vi "scan_operation.vi"(4 "Iter Counter In":u16[](array[numeric]), 5 "Prev DIO State":bool[](array[boolean])=[FALSE, FALSE, FALSE, FALSE, FALSE, FALSE, FALSE, FALSE, FALSE, FALSE, FALSE, FALSE, FALSE, FALSE, FALSE, FALSE, FALSE, FALSE, FALSE, FALSE, FALSE, FALSE, FALSE, FALSE, FALSE, FALSE, FALSE, FALSE, FALSE, FALSE, FALSE, FALSE], 6 "Digital Input Value Array":bool[](array[boolean])=[FALSE, FALSE, FALSE, FALSE, FALSE, FALSE, FALSE, FALSE, FALSE, FALSE, FALSE, FALSE, FALSE, FALSE, FALSE, FALSE, FALSE, FALSE, FALSE, FALSE, FALSE, FALSE, FALSE, FALSE, FALSE, FALSE, FALSE, FALSE, FALSE, FALSE, FALSE, FALSE], 7 "Channel":T1={"Operation"=0, "Num. Steps"=0, "Begin"=0.0, "Step Size"=0.0, "Input - A"=0, "Input - B"=0, "Output - LO"=0.0, "Output - HI"=0.0, "Reset"=FALSE, "Analog Output"=0, "Trigger Input"=0, "Initialize To"=0, "Digital Inputs"=[0, 0, 0, 0, 0], "Output Values"=[0.0, 0.0, 0.0, 0.0, 0.0], "Num. Inputs"=4} {"Digital Inputs" items=["DIO0", "DIO1", "DIO2", "DIO3", "DIO4", "DIO5", "DIO6", "DIO7", "DIO8", "DIO9", "DIO10", "DIO11", "DIO12", "DIO13", "DIO14", "DIO15", "DIO16", "DIO17", "DIO18", "DIO19", "DIO20", "DIO21", "DIO22", "DIO23", "DIO24", "DIO25", "DIO26", "DIO27", "DIO28", "DIO29", "DIO30", "DIO31"]; "Initialize To" items=["Zero", "Begin Value"]; "Trigger Input" items=["DIO0", "DIO1", "DIO2", "DIO3", "DIO4", "DIO5", "DIO6", "DIO7", "DIO8", "DIO9", "DIO10", "DIO11", "DIO12", "DIO13", "DIO14", "DIO15", "DIO16", "DIO17", "DIO18", "DIO19", "DIO20", "DIO21", "DIO22", "DIO23", "DIO24", "DIO25", "DIO26", "DIO27", "DIO28", "DIO29", "DIO30", "DIO31"]; "Analog Output" items=["AO\\00", "AO\\01", "AO\\02", "AO\\03", "AO\\04", "AO\\05", "AO\\06", "AO\\07", "AO\\08", "AO\\09", "AO\\10", "AO\\11", "AO\\12", "AO\\13", "AO\\14", "AO\\15"]; "Input - B" items=["DIO0", "DIO1", "DIO2", "DIO3", "DIO4", "DIO5", "DIO6", "DIO7", "DIO8", "DIO9", "DIO10", "DIO11", "DIO12", "DIO13", "DIO14", "DIO15", "DIO16", "DIO17", "DIO18", "DIO19", "DIO20", "DIO21", "DIO22", "DIO23", "DIO24", "DIO25", "DIO26", "DIO27", "DIO28", "DIO29", "DIO30", "DIO31"]; "Input - A" items=["DIO0", "DIO1", "DIO2", "DIO3", "DIO4", "DIO5", "DIO6", "DIO7", "DIO8", "DIO9", "DIO10", "DIO11", "DIO12", "DIO13", "DIO14", "DIO15", "DIO16", "DIO17", "DIO18", "DIO19", "DIO20", "DIO21", "DIO22", "DIO23", "DIO24", "DIO25", "DIO26", "DIO27", "DIO28", "DIO29", "DIO30", "DIO31"]; "Operation" items=["OFF", "SWITCH", "AND GATE", "OR GATE", "ITERATION", "CUSTOM - 461nm Freq."]}) -> (0 "Iter Counter Out":u16[](array[numeric]), 1 "Current DIO State":bool[](array[boolean]), 3 "AO out":fxp<+/-,20,5>)   [LabVIEW 2016]
uses:
  fpga_array_element.ctl
panel:
  # "Boolean Operation Controls"
  # "Iteration Operation Controls"
  # "Custom Operation Controls"
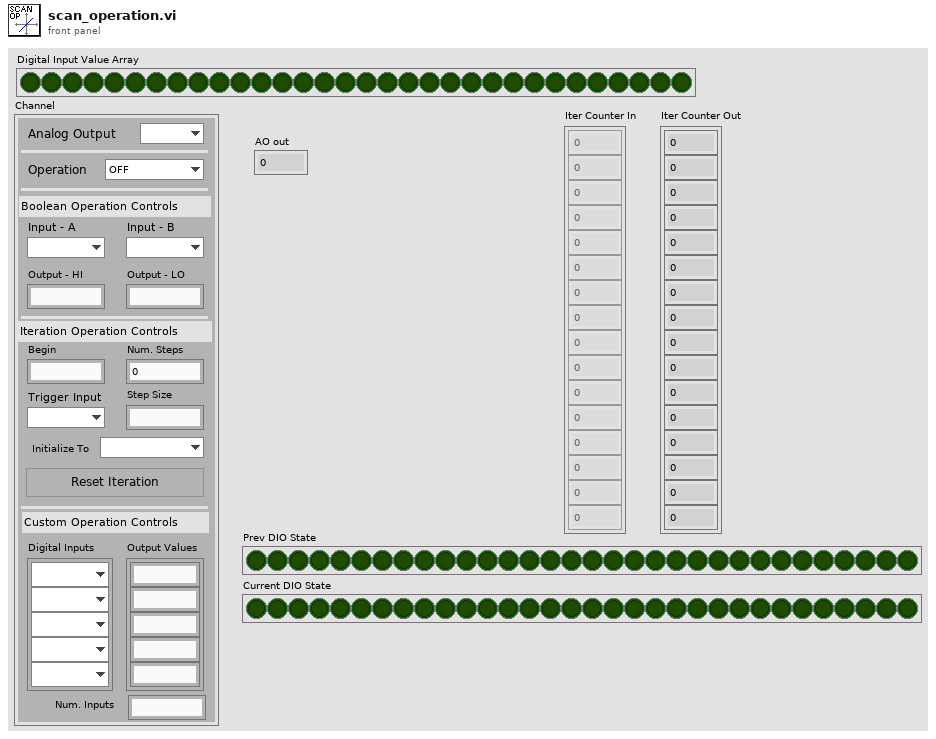
[diagram p1: front panel]
types:
  T1 = typedef "fpga_array_element.ctl" = cluster{"Operation":i16, "Num. Steps":u16, "Begin":fxp<+/-,20,5>, "Step Size":fxp<+/-,20,5>, "Input - A":i32, "Input - B":i32, "Output - LO":fxp<+/-,20,5>, "Output - HI":fxp<+/-,20,5>, "Reset":bool, "Analog Output":i32, "Trigger Input":i32, "Initialize To":i16, "Digital Inputs":i32[], "Output Values":fxp<+/-,20,5>[], "Num. Inputs":u16}
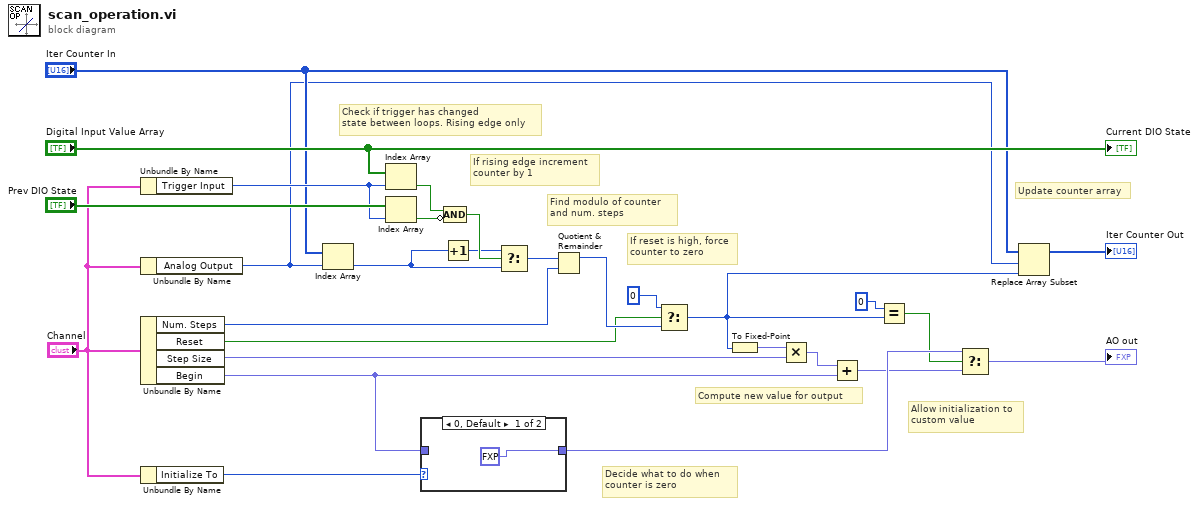
[diagram p0: block diagram]
diagram:
  # "Decide what to do when \ncounter is zero"
  # "Allow initialization to\ncustom value"
  # "Compute new value for output"
  # "Update counter array"
  # "If reset is high, force\ncounter to zero"
  # "Find modulo of counter\nand num. steps"
  # "If rising edge increment\ncounter by 1"
  # "Check if trigger has changed \nstate between loops. Rising edge only"
  n1 = Unbundle By Name("Channel") -> ("Trigger Input"=w24:i32)
  n2 = Unbundle By Name("Channel") -> ("Analog Output"=w1:i32)
  n3 = Unbundle By Name("Channel") -> ("Num. Steps"=w18:u16, "Reset"=w15:bool, "Step Size"=w14:fxp<+/-,20,5>, "Begin"=w10:fxp<+/-,20,5>)
  n4 = Unbundle By Name("Channel") -> ("Initialize To"=w11:i16)
  n5 = Index Array(array="Iter Counter In", index=w1) -> (element=w19:u16)
  n6 = Index Array(array="Digital Input Value Array", index=w24) -> (element=w26:bool)
  n7 = Index Array(array="Prev DIO State", index=w24) -> (element=w23:bool)
  n8 = case shown="0, Default" w11 {
    tunnel: w10 -> [_ w30]
    tunnel: [fxp<+/-,20,5> 0.0 w30] -> w7
    frame 0, Default {
    }
    frame 1 {
    }
  }
  n9 = Increment(x=w19) -> (x+1=w20:u16)
  n10 = Compound Arithmetic op=AND(w26, invert w23) -> (w28:bool)
  n11 = Select(t=w20, s=w28, f=w19) -> (s? t:f=w17:u16)
  n12 = Quotient & Remainder(x=w17, y=w18) -> (x-y*floor(x/y)=w16:u16)  [unwired: 1 out]
  n13 = Select(t=u16 0, s=w15, f=w16) -> (s? t:f=w9:u16)
  n14 = To Fixed-Point(number=w9) -> (fixed-point=w13:fxp<+/-,20,5>)  [unwired: 1 in]
  n15 = Multiply(x=w13, y=w14) -> (x*y=w12:fxp<+/-,40,10>)
  n16 = Add(x=w12, y=w10) -> (x+y=w6:fxp<+/-,40,10>)
  n17 = Equal?(x=u16 0, y=w9) -> (x = y?=w5:bool)
  n18 = Select(t=w7, s=w5, f=w6) -> (s? t:f=→"AO out":fxp<+/-,40,10>)
  n19 = Replace Array Subset(array="Iter Counter In", new element=w9, index=w1) -> (→"Iter Counter Out":u16[])
  "Current DIO State" <- "Digital Input Value Array"
